vi "Change Read Directory.vi"(8 "error in":errorcluster, 10 "file directory":path, 11 "node":refnum<class "module editor node.lvclass">) -> (0 "error out":errorcluster, 3 "node out":refnum<class "module editor node.lvclass">)   [LabVIEW 2013, in "Shared Memory Editor Node.lvclass"]
uses:
  Shared Memory Editor Node.lvclass
  <vilib>/NI/Tag Bus Data Framework/Configuration Editor/Classes/Module editor node/module editor node.lvclass
  module/configuration/Shared Memory Configuration.lvclass
  <vilib>/NI/Configuration Framework/serializable configuration/NISE_CEF_serializable configuration.lvclass
  module/configuration/Shared Memory Configuration.lvclass/Shared Memory Configuration.ctl
  module/configuration/Write Read Directory.vi
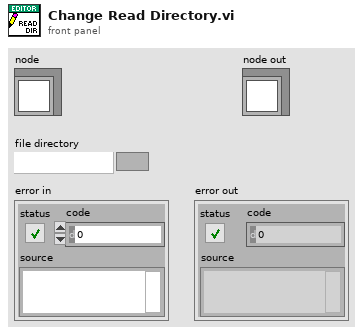
[diagram p1: front panel]
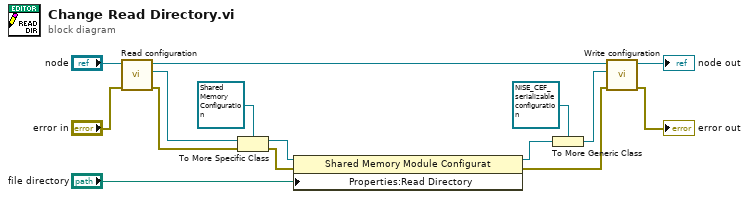
[diagram p0: block diagram]
diagram:
  n1 = call-dynamic "Read configuration.vi"("error in"="error in", "NISE_CEF_serializable node in"="node") -> ("error out"=w4:errorcluster, "configuration"=w8:refnum<class "NISE_CEF_serializable configuration.lvclass">, "NISE_CEF_serializable node out"=w6:refnum<class "module editor node.lvclass">)  [unwired: 7 in]
  n2 = To More Specific Class(target class=refnum<class "Shared Memory Configuration.lvclass"> refnum ("Shared Memory Configuration out"), reference=w8, error in=w4) -> (specific class reference=w7:refnum<class "Shared Memory Configuration.lvclass">, error out=w14:errorcluster)
  n3 = property class="Shared Memory Module Configurat"(reference=w7, error in=w14, "Properties:Read Directory"="file directory") -> (reference out=w11:refnum<class "Shared Memory Configuration.lvclass">, error out=w3:errorcluster)
  n4 = To More Generic Class(target class=refnum<class "NISE_CEF_serializable configuration.lvclass"> refnum ("configuration"), reference=w11) -> (generic class reference=w12:refnum<class "NISE_CEF_serializable configuration.lvclass">)
  n5 = call-dynamic "Write configuration.vi"("error in"=w3, "configuration"=w12, "NISE_CEF_serializable node in"=w6) -> ("error out"=→"error out":errorcluster, "NISE_CEF_serializable node out"=→"node out":refnum<class "module editor node.lvclass">)  [unwired: 7 in]
